vi "Run Bfr Rx - Handle Rollover.vi"(7 "Offset in":u64, 8 "error in (no error)":errorcluster, 10 "Data in":u8[](array[numeric]), 11 "Buffer Size":u64) -> (0 "error out":errorcluster, 2 "Rollover?":bool, 5 "Offset out":u64)   [LabVIEW 2019, in "UDP-Custom-Device Engine.lvlib"]
uses:
  UDP-Custom-Device Engine.lvlib
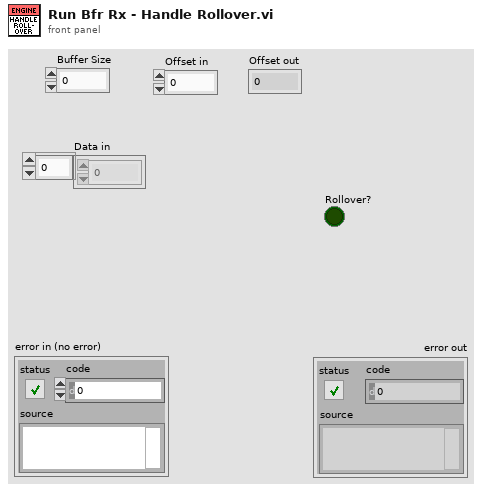
[diagram p1: front panel]
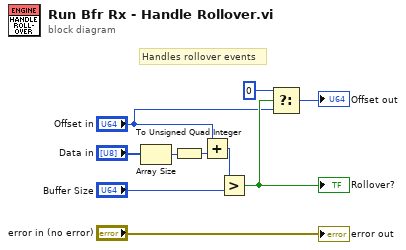
[diagram p0: block diagram]
diagram:
  # "Handles rollover events"
  n1 = Array Size(array="Data in") -> (size(s)=w9:i32)
  n2 = To Unsigned Quad Integer(1:w9) -> (0:w1:u64)
  n3 = Add(x="Offset in", y=w1) -> (x+y=w8:u64)
  n4 = Greater?(x=w8, y="Buffer Size") -> (0:w6:bool)
  "Rollover?" <- w6
  n5 = Select(t=u64 0, s=w6, f="Offset in") -> (s? t:f=→"Offset out":u64)
  "error out" <- "error in (no error)"
